vi "ADC Test.vi"() -> ()   [LabVIEW 2019]
panel:
  out "mean":dbl format="%0.2f"
  out "error out":errorcluster
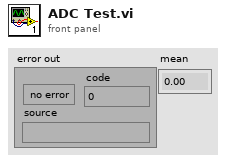
[diagram p1: front panel]
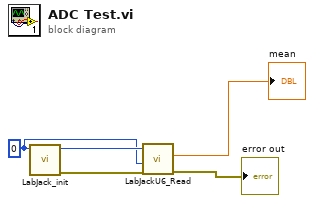
[diagram p0: block diagram]
diagram:
  w1 = 0 ("Positive Channel #")
  n1 = call "LabJack_init.vi"("Positive Channel #"=w1) -> ("error out"=w5:errorcluster, "Handle Out"=w4:i32)  [unwired: 8 in, 1 out]
  n2 = call "LabJackU6_Read.vi"("error in"=w5, "Positive Channel #"=w1, "Handle In"=w4) -> ("error out"=→"error out":errorcluster, "mean"=→"mean":dbl)  [unwired: 6 in, 1 out]
